vi "Robo Team Send Stream Command.vi"(5 "Action":enum16{"At End", "At Front"}(ring), 7 "timeout in ms (0)":i32, 8 "error in (no error)":errorcluster, 10 "Data in":variant, 11 "Command":string) -> (0 "error out":errorcluster, 2 "Data out":variant)   [LabVIEW 2015]
uses:
  Robo Team Engine Command.ctl
  Robo Team Globals.vi
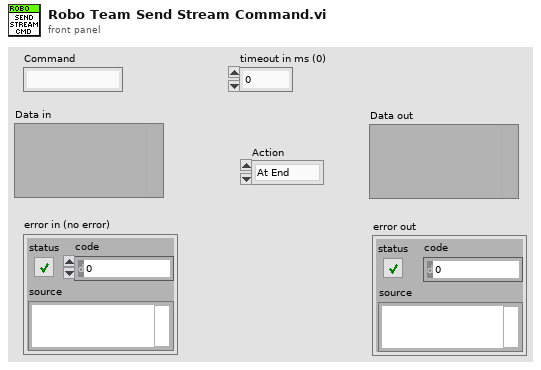
[diagram p1: front panel]
types:
  T1 = typedef "Robo Team Engine Command.ctl" = cluster{"Command":string, "Data":variant, "Error":errorcluster, "Timeout":i32}
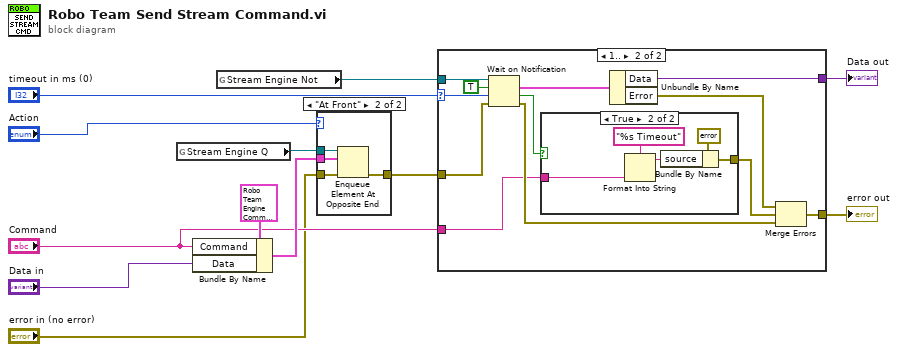
[diagram p0: block diagram]
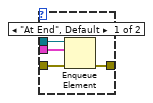
[diagram p4: hidden frame]
diagram:
  n1 = global read "Robo Team Globals.vi" "Stream Engine Q"() -> (w6:refnum<queue>)
  n2 = Bundle By Name(cluster=T1 {"Command"="", "Data"=variant, "Error"={"status"=FALSE, "code"=0, "source"=""}, "Timeout"=0} ("element"), "Command"="Command", "Data"="Data in") -> (w10:T1)
  n3 = global read "Robo Team Globals.vi" "Stream Engine Not"() -> (w7:refnum<notifier>)
  n4 = case shown="\"At Front\"" "Action" {
    tunnel: w10 -> [w16 w17]
    tunnel: [w15 w18] -> w8
    tunnel: w6 -> [w14 w20]
    tunnel: "error in (no error)" -> [w13 w19]
    frame "At End", Default {
      n5 = Enqueue Element(queue=w14, element=w16, error in (no error)=w13) -> (error out=w15:errorcluster)  [unwired: 1 in, 2 out]
    }
    frame "At Front" {
      n6 = Enqueue Element At Opposite End(queue=w20, element=w17, error in (no error)=w19) -> (error out=w18:errorcluster)  [unwired: 1 in, 2 out]
    }
  }
  n7 = case shown="1.." "timeout in ms (0)" {
    selector: "timeout in ms (0)" -> [_ w21]
    tunnel: [_ w32] -> w11
    tunnel: w8 -> [_ w29]
    tunnel: w7 -> [_ w28]
    tunnel: [_ w26] -> w5
    tunnel: "Command" -> [_ w22]
    frame 0, Default {
    }
    frame 1.. {
      n8 = Wait on Notification(notifier=w28, ignore previous (F)=TRUE, timeout in ms (-1)=w21, error in (no error)=w29) -> (notification=w31:T1, timed out?=w25:bool, error out=w27:errorcluster)  [unwired: 1 out]
      n9 = case shown="True" w25 {
        tunnel: [_ w36] -> w23
        tunnel: w22 -> [_ w33]
        frame False {
        }
        frame True {
          n10 = Format Into String(format string="%s Timeout", w33) -> (resulting string=w35:string)  [unwired: 2 in, 1 out]
          n11 = Bundle By Name(cluster=errorcluster {"status"=TRUE, "code"=5001, "source"=""} ("Error"), "source"=w35) -> (w36:errorcluster)
        }
      }
      n12 = Unbundle By Name(w31) -> ("Data"=w32:variant, "Error"=w24:errorcluster)
      n13 = Merge Errors(w24, w23, w27) -> (w26:errorcluster)
    }
  }
  "error out" <- w5
  "Data out" <- w11
